vi "Records Assert Equal.vi"(7 "Assertion Label":string, 8 "Error In":errorcluster, 9 "Correct Records":refnum<class "Expenses Tracker Record.lvclass">[](array[class]), 10 "Typedef Records":variant[](array[variant]), 11 "Expenses Tracker Record In":refnum<class "Expenses Tracker Record.lvclass">) -> (0 "Error Out":errorcluster)   [LabVIEW 2023]
uses:
  <vilib>/addons/_JKI Toolkits/Caraya/classes/Assert/Assert.lvclass
  <vilib>/addons/_JKI Toolkits/Caraya/classes/Assert/Assert Equal Value_Variant.vi
  Interfaces/Expenses Tracker Record/Expenses Tracker Record.lvclass
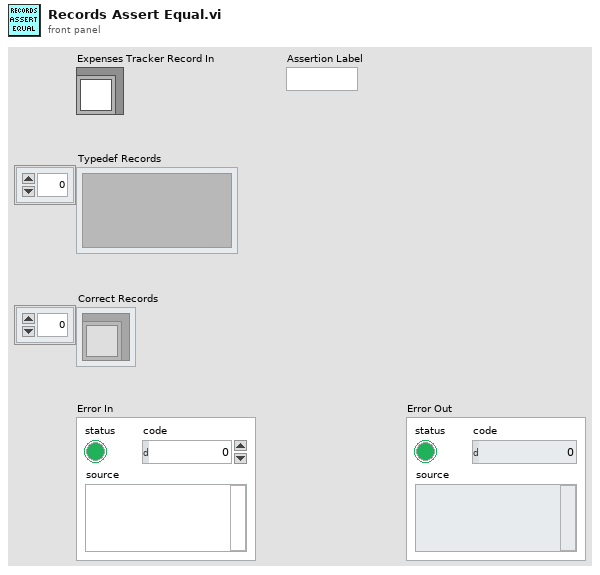
[diagram p1: front panel]
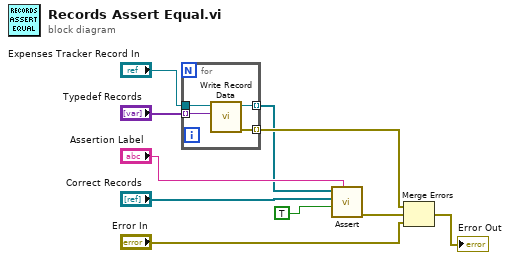
[diagram p0: block diagram]
diagram:
  n1 = for {
    tunnel: "Typedef Records" -> [w14] mode=indexing
    tunnel: "Expenses Tracker Record In" -> [w13]
    tunnel: [w12] -> w4 mode=indexing
    tunnel: [w11] -> w7 mode=indexing
    n2 = call-dynamic "Write Record Data.vi"("Record"=w14, "Expenses Tracker Record In"=w13) -> ("Error Out"=w11:errorcluster, "Expenses Tracker Record Out"=w12:refnum<class "Expenses Tracker Record.lvclass">)  [unwired: 8 in]
  }
  n3 = call-poly <vilib>:"Assert.vi"("Label"="Assertion Label", "Register with caller test (F)"=TRUE, "Y"="Correct Records", "X"=w4) -> ("error out"=w2:errorcluster)  [unwired: 6 in, 1 out]
  n4 = Merge Errors(w7, w2, "Error In") -> (→"Error Out":errorcluster)
